vi "dataconv.vi"(11 "Array":sgl[](array[numeric])) -> (1 "n":i32, 2 "WH":sgl[][](array[numeric]), 3 "XY":sgl[][](array[numeric]))   [LabVIEW 2020]
panel:
  out "output array":dbl[][](array[numeric])
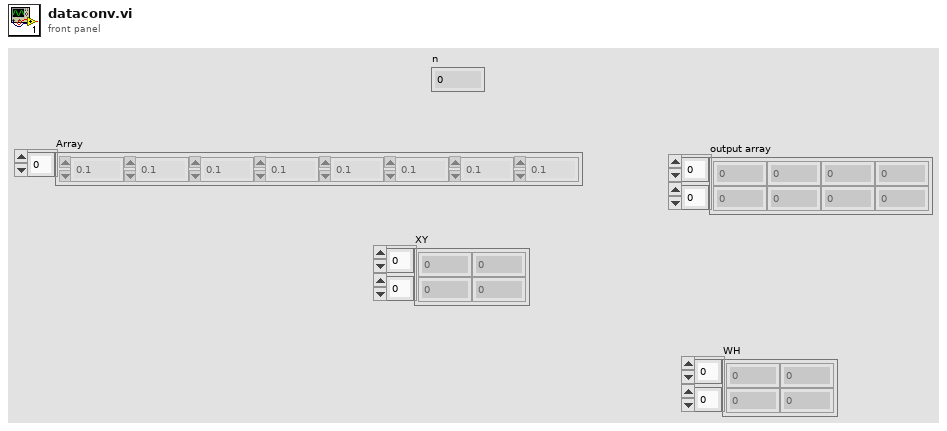
[diagram p1: front panel]
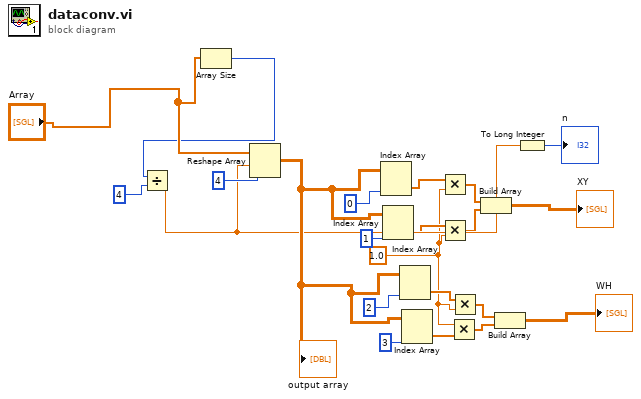
[diagram p0: block diagram]
diagram:
  w3 = 1.0
  n1 = Array Size(array="Array") -> (size(s)=w20:i32)
  n2 = Divide(x=w20, y=4 ("dimension size")) -> (x/y=w11:dbl)
  n3 = Reshape Array("Array", w11, 4 ("dimension size")) -> (w12:sgl[][])
  "output array" <- w12
  n4 = Index Array(array=w12, index (col)=0 ("disabled index (col)")) -> (element=w9:sgl[])  [unwired: 1 in]
  n5 = Index Array(array=w12, index (col)=1 ("disabled index (col)")) -> (element=w7:sgl[])  [unwired: 1 in]
  n6 = Index Array(array=w12, index (col)=2 ("disabled index (col)")) -> (element=w4:sgl[])  [unwired: 1 in]
  n7 = Index Array(array=w12, index (col)=3 ("disabled index (col)")) -> (element=w5:sgl[])  [unwired: 1 in]
  n8 = Multiply(x=w9, y=w3) -> (x*y=w8:dbl[])
  n9 = Multiply(x=w7, y=w3) -> (x*y=w6:dbl[])
  n10 = Multiply(x=w3, y=w5) -> (x*y=w1:dbl[])
  n11 = Multiply(x=w4, y=w3) -> (x*y=w2:dbl[])
  n12 = Build Array(w8, w6) -> (→"XY":dbl[][])
  n13 = Build Array(w2, w1) -> (→"WH":dbl[][])
  n14 = To Long Integer(number=w11) -> (32bit integer=→"n":i32)
